vi "Vary Frequency Continuous with Disc Waveform.vi"() -> ()   [LabVIEW 2020]
uses:
  <vilib>/DAQmx/write.llb/DAQmx Write (Analog Wfm 1Chan NSamp).vi
  <vilib>/DAQmx/create/channels.llb/DAQmx Create Channel (AO-Voltage-Basic).vi
  <vilib>/DAQmx/configure/timing.llb/DAQmx Timing (Use Waveform).vi
  <vilib>/DAQmx/miscellaneous.llb/DAQmx Fill In Error Info.vi
  <vilib>/measure/NI_MABase.lvlib
panel:
  in  "Dual Sources?":bool
  out "Waveform Chart":waveform(dbl)(graph)
  in  "DAQmx Physical Channel":tag
  in  "Blocking Waveform Selection":T1(tab)
  in  "Waveform Type":T2(ring)
  in  "Full Pulse\nWidth (us)":dbl=10.0 min=10.0 step=2.0
  in  "stop":bool
  in  "Waveform\nAmplitude (mApp)":dbl
  in  "Waveform\nFrequency (Hz)":i64=1 min=1 max=100000 step=1
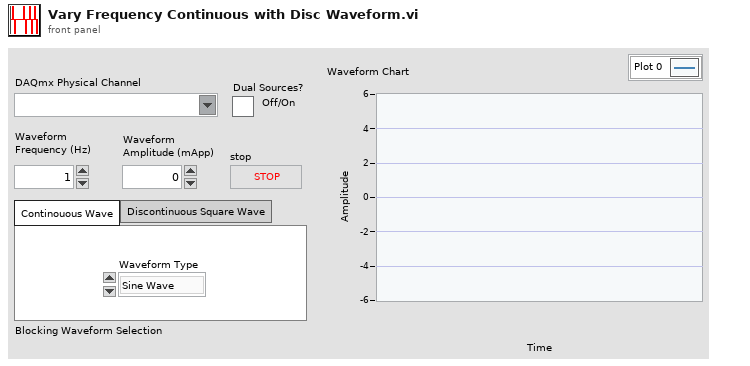
[diagram p1: front panel]
types:
  T1 = enum32{"Continouous Wave", "Discontinuous Square Wave"}
  T2 = enum16{"Sine Wave", "Triangle Wave", "Square Wave", "Sawtooth Wave"}
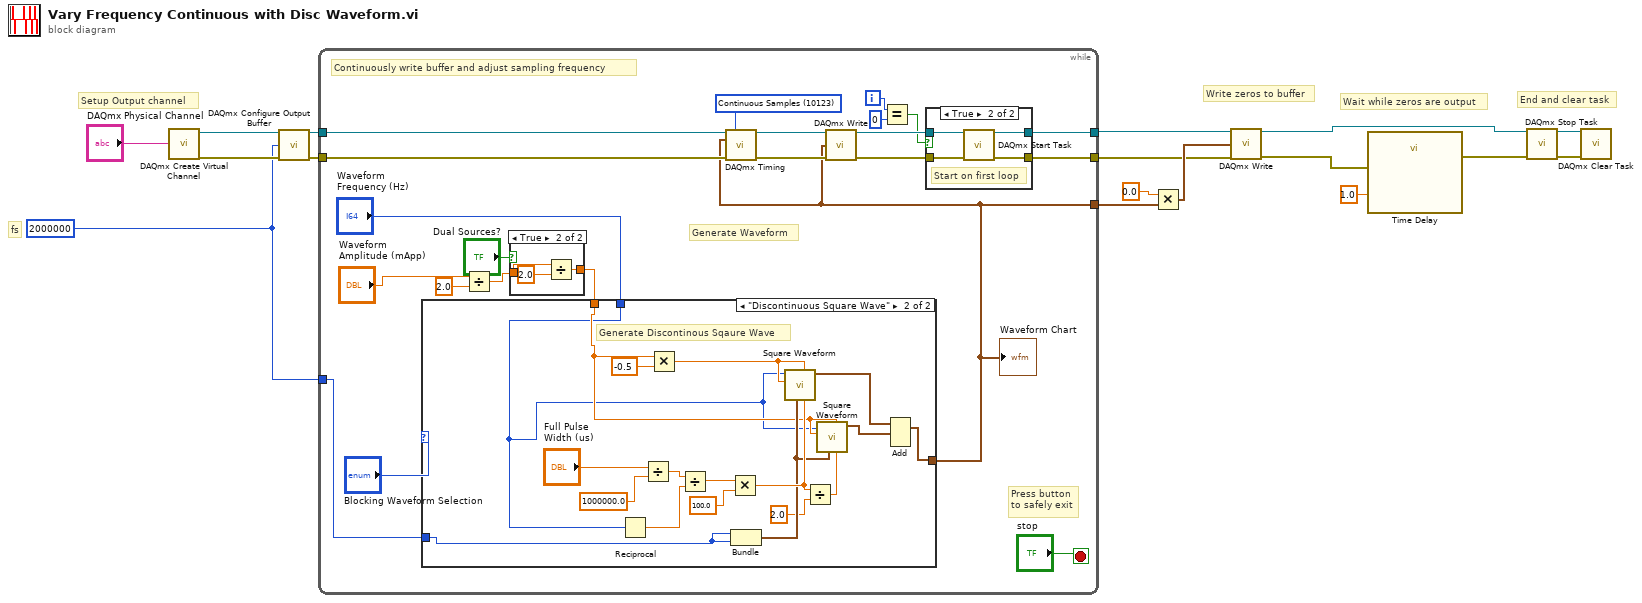
[diagram p0: block diagram]
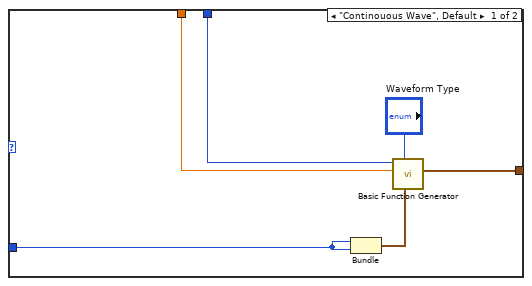
[diagram p3: hidden frame]
diagram:
  w2 = 2000000
  # "fs"
  # "End and clear task"
  # "Wait while zeros are output"
  # "Write zeros to buffer"
  # "Setup Output channel"
  n1 = call-poly <vilib>:"DAQmx Create Virtual Channel.vi"("physical channels"="DAQmx Physical Channel") -> ("task out"=w16:refnum<k21>, "error out"=w17:errorcluster)  [unwired: 13 in]
  n2 = call <vilib>:"DAQmx Configure Output Buffer.vi"("task/channels in"=w16, "buffer size (in samples per channel)"=w2, "error in"=w17) -> ("task out"=w15:refnum<k21>, "error out"=w14:errorcluster)  [unwired: 11 in]
  n3 = while {
    tunnel: w15 -> [w39]
    tunnel: w14 -> [w38]
    tunnel: w2 -> [w24]
    tunnel: [w33] -> w6
    tunnel: [w23] -> w9
    tunnel: [w27] -> w5
    i -> [w29]
    stop <- "stop" stop-if-true
    w31 = 10123 items=["Finite Samples"=10178, "Continuous Samples"=10123, "Hardware Timed Single Point"=12522] ("sample mode")
    # "Press button\nto safely exit"
    # "Generate Waveform"
    # "Continuously write buffer and adjust sampling frequency"
    n4 = Divide(x="Waveform\nAmplitude (mApp)", y=2.0) -> (x/y=w20:dbl)
    n5 = case shown="True" "Dual Sources?" {
      tunnel: w20 -> [w40 w42]
      tunnel: [w40 w41] -> w18
      frame False {
      }
      frame True {
        n6 = Divide(x=w42, y=2.0) -> (x/y=w41:dbl)
      }
    }
    n7 = case shown="\"Discontinuous Square Wave\"" "Blocking Waveform Selection" {
      tunnel: "Waveform\nFrequency (Hz)" -> [w46 w52]
      tunnel: w24 -> [w45 w51]
      tunnel: w18 -> [w47 w53]
      tunnel: [w44 w50] -> w23
      frame "Continouous Wave", Default {
        n8 = Bundle(w45, w45) -> (w49:cluster{i32, i32})  [unwired: 1 in]
        n9 = call <vilib>:"Basic Function Generator.vi"("sampling info"=w49, "signal type"="Waveform Type", "amplitude"=w47, "frequency"=w46) -> ("signal out"=w44:waveform(dbl))  [unwired: 5 in, 2 out]
      }
      frame "Discontinuous Square Wave" {
        # "Generate Discontinous Sqaure Wave"
        n10 = Reciprocal(x=w52) -> (1/x=w63:dbl)
        n11 = Divide(x="Full Pulse\nWidth (us)", y=1000000.0) -> (x/y=w65:dbl)
        n12 = Multiply(x=w53, y=-0.5) -> (x*y=w60:dbl)
        n13 = Divide(x=w65, y=w63) -> (x/y=w67:dbl)
        n14 = Multiply(x=w67, y=100.0) -> (x*y=w66:dbl)
        n15 = Bundle(w51, w51) -> (w62:cluster{i32, i32})  [unwired: 1 in]
        n16 = call <vilib>:"Square Waveform.vi"("duty cycle (%)"=w66, "offset"=w60, "sampling info"=w62, "amplitude"=w60, "frequency"=w52) -> ("signal out"=w58:waveform(dbl))  [unwired: 5 in, 1 out]
        n17 = Divide(x=w66, y=2.0) -> (x/y=w61:dbl)
        n18 = call <vilib>:"Square Waveform.vi"("duty cycle (%)"=w61, "offset"=w53, "sampling info"=w62, "amplitude"=w53, "frequency"=w52) -> ("signal out"=w59:waveform(dbl))  [unwired: 5 in, 1 out]
        n19 = Add(1:w59, 2:w58) -> (0:w50:waveform(dbl))  [unwired: 1 in, 1 out]
      }
    }
    "Waveform Chart" <- w23
    n20 = call-poly <vilib>:"DAQmx Timing.vi"("task/channels in"=w39, "sample mode"=w31, "waveform"=w23, "error in"=w38) -> ("task out"=w37:refnum<k21>, "error out"=w36:errorcluster)  [unwired: 10 in]
    n21 = call-poly <vilib>:"DAQmx Write.vi"("task/channels in"=w37, "data"=w23, "error in"=w36) -> ("task out"=w35:refnum<k21>, "error out"=w34:errorcluster)  [unwired: 10 in, 1 out]
    n22 = Equal?(x=w29, y=0) -> (x = y?=w30:bool)
    n23 = case shown="True" w30 {
      tunnel: w35 -> [w69 w73]
      tunnel: w34 -> [w68 w72]
      tunnel: [w69 w71] -> w33
      tunnel: [w68 w70] -> w27
      frame False {
      }
      frame True {
        # "Start on first loop"
        n24 = call <vilib>:"DAQmx Start Task.vi"("task/channels in"=w73, "error in"=w72) -> ("task out"=w71:refnum<k21>, "error out"=w70:errorcluster)  [unwired: 12 in]
      }
    }
  }
  n25 = Multiply(x=0.0, y=w9) -> (x*y=w7:waveform(dbl))
  n26 = call-poly <vilib>:"DAQmx Write.vi"("task/channels in"=w6, "data"=w7, "error in"=w5) -> ("task out"=w8:refnum<k21>, "error out"=w4:errorcluster)  [unwired: 10 in, 1 out]
  n27 = call "Time Delay"("error in (no error)"=w4, "Delay Time (s)"=1.0) -> ("error out"=w3:errorcluster)  [unwired: 9 in]
  n28 = call <vilib>:"DAQmx Stop Task.vi"("task/channels in"=w8, "error in"=w3) -> ("task out"=w13:refnum<k21>, "error out"=w12:errorcluster)  [unwired: 12 in]
  n29 = call <vilib>:"DAQmx Clear Task.vi"("task in"=w13, "error in"=w12) -> ()  [unwired: 13 in, 1 out]
